vi "CreateTopLevelDiagram.vi"(8 "error in":errorcluster, 11 "PythonConverter_BD in":refnum<class "PyConvBD.lvclass">) -> (0 "error out":errorcluster, 3 "PythonConverter_BD out":refnum<class "PyConvBD.lvclass">)   [LabVIEW 2014, in "Raspberry Pi Compatible Compiler for LabVIEW.lvlib" / "PyConvBD.lvclass"]
uses:
  PyConvBD.lvclass
  PyConvBD.lvclass/PyConvBD.ctl
  VI Interpreter/Classes/TopLevelDiagram/TopLevelDiagram.lvclass
  VI Interpreter/Classes/VI Interpreter/VI Interpreter.lvclass
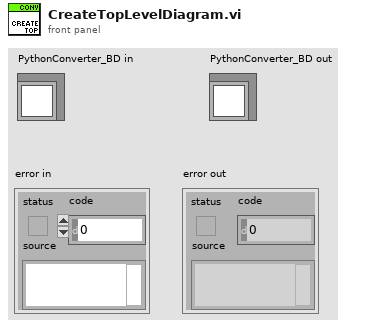
[diagram p1: front panel]
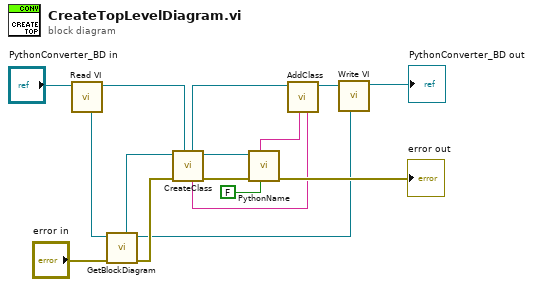
[diagram p0: block diagram]
diagram:
  n1 = call "Read VI.vi"("PythonConverter_BD in"="PythonConverter_BD in") -> ("PythonConverter_BD out"=w9:refnum<class "PyConvBD.lvclass">, "VI Interpreter"=w8:refnum<class "VI Interpreter.lvclass">)  [unwired: 7 in]
  n2 = call "GetBlockDiagram.vi"("error in"="error in", "VI Interpreter in"=w8) -> ("error out"=w14:errorcluster, "VI Interpreter out"=w2:refnum<class "VI Interpreter.lvclass">, "TopLevelDiagram"=w13:refnum<class "TopLevelDiagram.lvclass">)  [unwired: 5 in]
  n3 = call-dynamic "CreateClass.vi"("PythonConverter_BD in"=w9, "error in"=w14, "Diagram in"=w13) -> ("error out"=w15:errorcluster, "Diagram out"=w12:refnum<class "TopLevelDiagram.lvclass">, "diagram"=w4:string, "PythonConverter_BD out"=w6:refnum<class "PyConvBD.lvclass">)  [unwired: 5 in]
  n4 = call-dynamic "PythonName.vi"("add self"=FALSE, "error in"=w15, "Diagram in"=w12) -> ("error out"=→"error out":errorcluster, "UID"=w5:string)  [unwired: 5 in, 2 out]
  n5 = call "AddClass.vi"("definition"=w4, "name"=w5, "PythonConverter_BD in"=w6) -> ("PythonConverter_BD out"=w3:refnum<class "PyConvBD.lvclass">)  [unwired: 5 in, 1 out]
  n6 = call "Write VI.vi"("VI Interpreter"=w2, "PythonConverter_BD in"=w3) -> ("PythonConverter_BD out"=→"PythonConverter_BD out":refnum<class "PyConvBD.lvclass">)  [unwired: 7 in]
